vi "1BS3HD_Tidy_v00.vi"(0 "Extras 1SDI":T1={"Error Bit Shift "={"EPR BS"=0, "HD A x"=0, "HD A p"=0, "HD B x"=0, "HD B p"=0, "HD C x"=0, "HD C p"=0}, "I Max value"=20000, "Scan Offset"={"EPR BS"=0.0, "HD A"=0.0, "HD B"=0.0, "HD C"=0.0}, "Scan Ampl.\n     (mV)"={"EPR BS"=0.0, "HD A"=0.0, "HD B"=0.0, "HD C"=0.0}, "Scan-PII thresh"={"EPR BS"=0, "Homodyne A"=0, "Homodyne B"=0, "Homodyne C"=0}, "Re-Scan thresh"={"EPR BS"=1000, "Homodyne A"=1000, "Homodyne B"=1000, "Homodyne C"=0}, "Post-Offset"={"HD A x"=0.0, "HD A p"=0.0, "HD B x"=0.0, "HD B p"=0.0, "HD C x"=0.0, "HD C p"=0.0}}, 5 "EPR BS":T5={"Offset Error"=-0.0003333333333333334, "Gain Error"=1, "P Gain"=25, "P Bit Shift"=-10, "I Bit Shift"=-10, "I Gain"=23, "Lock Threshold"=22, "Lock"=FALSE, "Hold"=FALSE, "Scan Frequency"=17, "Scan Bit Shift"=-4, "Gains +/- "=FALSE, "Pre- Offset Error"=0.0005084745762711861} {"Pre- Offset Error" scale=-0.01..0.01 scale format="%#_5f"; "Scan Frequency" scale=1.0..30.0; "I Gain" scale=0.0..50.0; "P Gain" scale=0.0..50.0; "Offset Error" scale=-0.01..0.01 scale format="%#_5f"}, 7 "Homodyne A":T13={"P Gain"=27, "P Bit Shift"=-8, "I Bit Shift"=-8, "I Gain"=19, "Lock Threshold"=37, "Lock"=FALSE, "Hold"=FALSE, "Scan Frequency"=13, "Scan Bit Shift"=-5, "Gains +/- "=FALSE, "Pre- Offset x"=0.0008474576271186437, "Pre-Offset p"=-0.0023163841807909607, "Gain Error x"=1, "Lock Angle"=0.0, "Gain Error p\n\n"=1} {"Lock Angle" min=-90.0 max=90.0 scale=-90.0..90.0 scale format="%#_2g"; "Pre-Offset p" scale=-0.01..0.01 scale format="%#_5f"; "Pre- Offset x" scale=-0.01..0.01 scale format="%#_5f"; "Scan Frequency" scale=1.0..30.0; "I Gain" scale=0.0..50.0; "P Gain" scale=0.0..50.0}, 9 "Homodyne B":T13={"P Gain"=14, "P Bit Shift"=-8, "I Bit Shift"=-8, "I Gain"=22, "Lock Threshold"=48, "Lock"=FALSE, "Hold"=FALSE, "Scan Frequency"=19, "Scan Bit Shift"=-5, "Gains +/- "=FALSE, "Pre- Offset x"=-0.0016384180790960455, "Pre-Offset p"=-0.002090395480225989, "Gain Error x"=1, "Lock Angle"=15.0, "Gain Error p\n\n"=1} {"Lock Angle" min=-90.0 max=90.0 scale=-90.0..90.0 scale format="%#_2g"; "Pre-Offset p" scale=-0.01..0.01 scale format="%#_5f"; "Pre- Offset x" scale=-0.01..0.01 scale format="%#_5f"; "Scan Frequency" scale=1.0..30.0; "I Gain" scale=0.0..50.0; "P Gain" scale=0.0..50.0}, 11 "Homodyne C":T13={"P Gain"=14, "P Bit Shift"=-8, "I Bit Shift"=-8, "I Gain"=22, "Lock Threshold"=48, "Lock"=FALSE, "Hold"=FALSE, "Scan Frequency"=19, "Scan Bit Shift"=-5, "Gains +/- "=FALSE, "Pre- Offset x"=-0.0016384180790960455, "Pre-Offset p"=-0.002090395480225989, "Gain Error x"=1, "Lock Angle"=15.0, "Gain Error p\n\n"=1} {"Lock Angle" min=-90.0 max=90.0 scale=-90.0..90.0 scale format="%#_2g"; "Pre-Offset p" scale=-0.01..0.01 scale format="%#_5f"; "Pre- Offset x" scale=-0.01..0.01 scale format="%#_5f"; "Scan Frequency" scale=1.0..30.0; "I Gain" scale=0.0..50.0; "P Gain" scale=0.0..50.0}, 12 "Hold All":T16, 14 "Scope+Safety":T18={"Safety First"={"lim reset"=FALSE, "no limit"=FALSE, "pos slew rate * dt"=100, "neg slew rate * dt"=-100, "Count(Ticks)"=0}, "Scope IPs"={"Trigger Direction"=enum."minus-plus", "Trigger Delay (ms)"=0.0, "Aquisition Rate (kHz)"=4000.0, "Trigger Offset (V)"=0.0, "Scale Offset"={"Scaling"={"Error signal"=1, "Output"=1, "DC Monitor"=1, "Threshold"=1}, "Offset"={"Error Signal"=0, "Output"=0, "DC Monitor"=0, "Threshold"=0}}}}) -> (4 "1SDI Control":T15)   [LabVIEW 2013]
doc: "The data structures from the User Interface need are rebundled here to match that of the FPGA_Cavity VI."
uses:
  Strict Type Defs/1BS3HD Control GUI HD.ctl
  Strict Type Defs/PII Gains.ctl
  Strict Type Defs/I16 white control.ctl
  Strict Type Defs/Thresh slider.ctl
  Strict Type Defs/Lock or Hold.ctl
  Strict Type Defs/Scan Freq Slider.ctl
  Strict Type Defs/Gains negative horizontal.ctl
  Strict Type Defs/Slider and display.ctl
  Strict Type Defs/theta 1SDI.ctl
  Strict Type Defs/1BS3HD Control GUI EPR.ctl
  Strict Type Defs/Scope and Safety.ctl
  Strict Type Defs/Safety First.ctl
  Strict Type Defs/Hold All.ctl
  Strict Type Defs/1BS3HD Control dummy.ctl
  Strict Type Defs/1BS3HD Lock Select.ctl
  Strict Type Defs/1BS3HD Extras.ctl
  Strict Type Defs/1BS3HD Double control.ctl
  Strict Type Defs/1BS3HD I16 Control.ctl
panel:
  in  "Lock Select":T4
  in  "1SDI Control dummy":T15
  in  "Safety First":T17
  # "Error Signal"
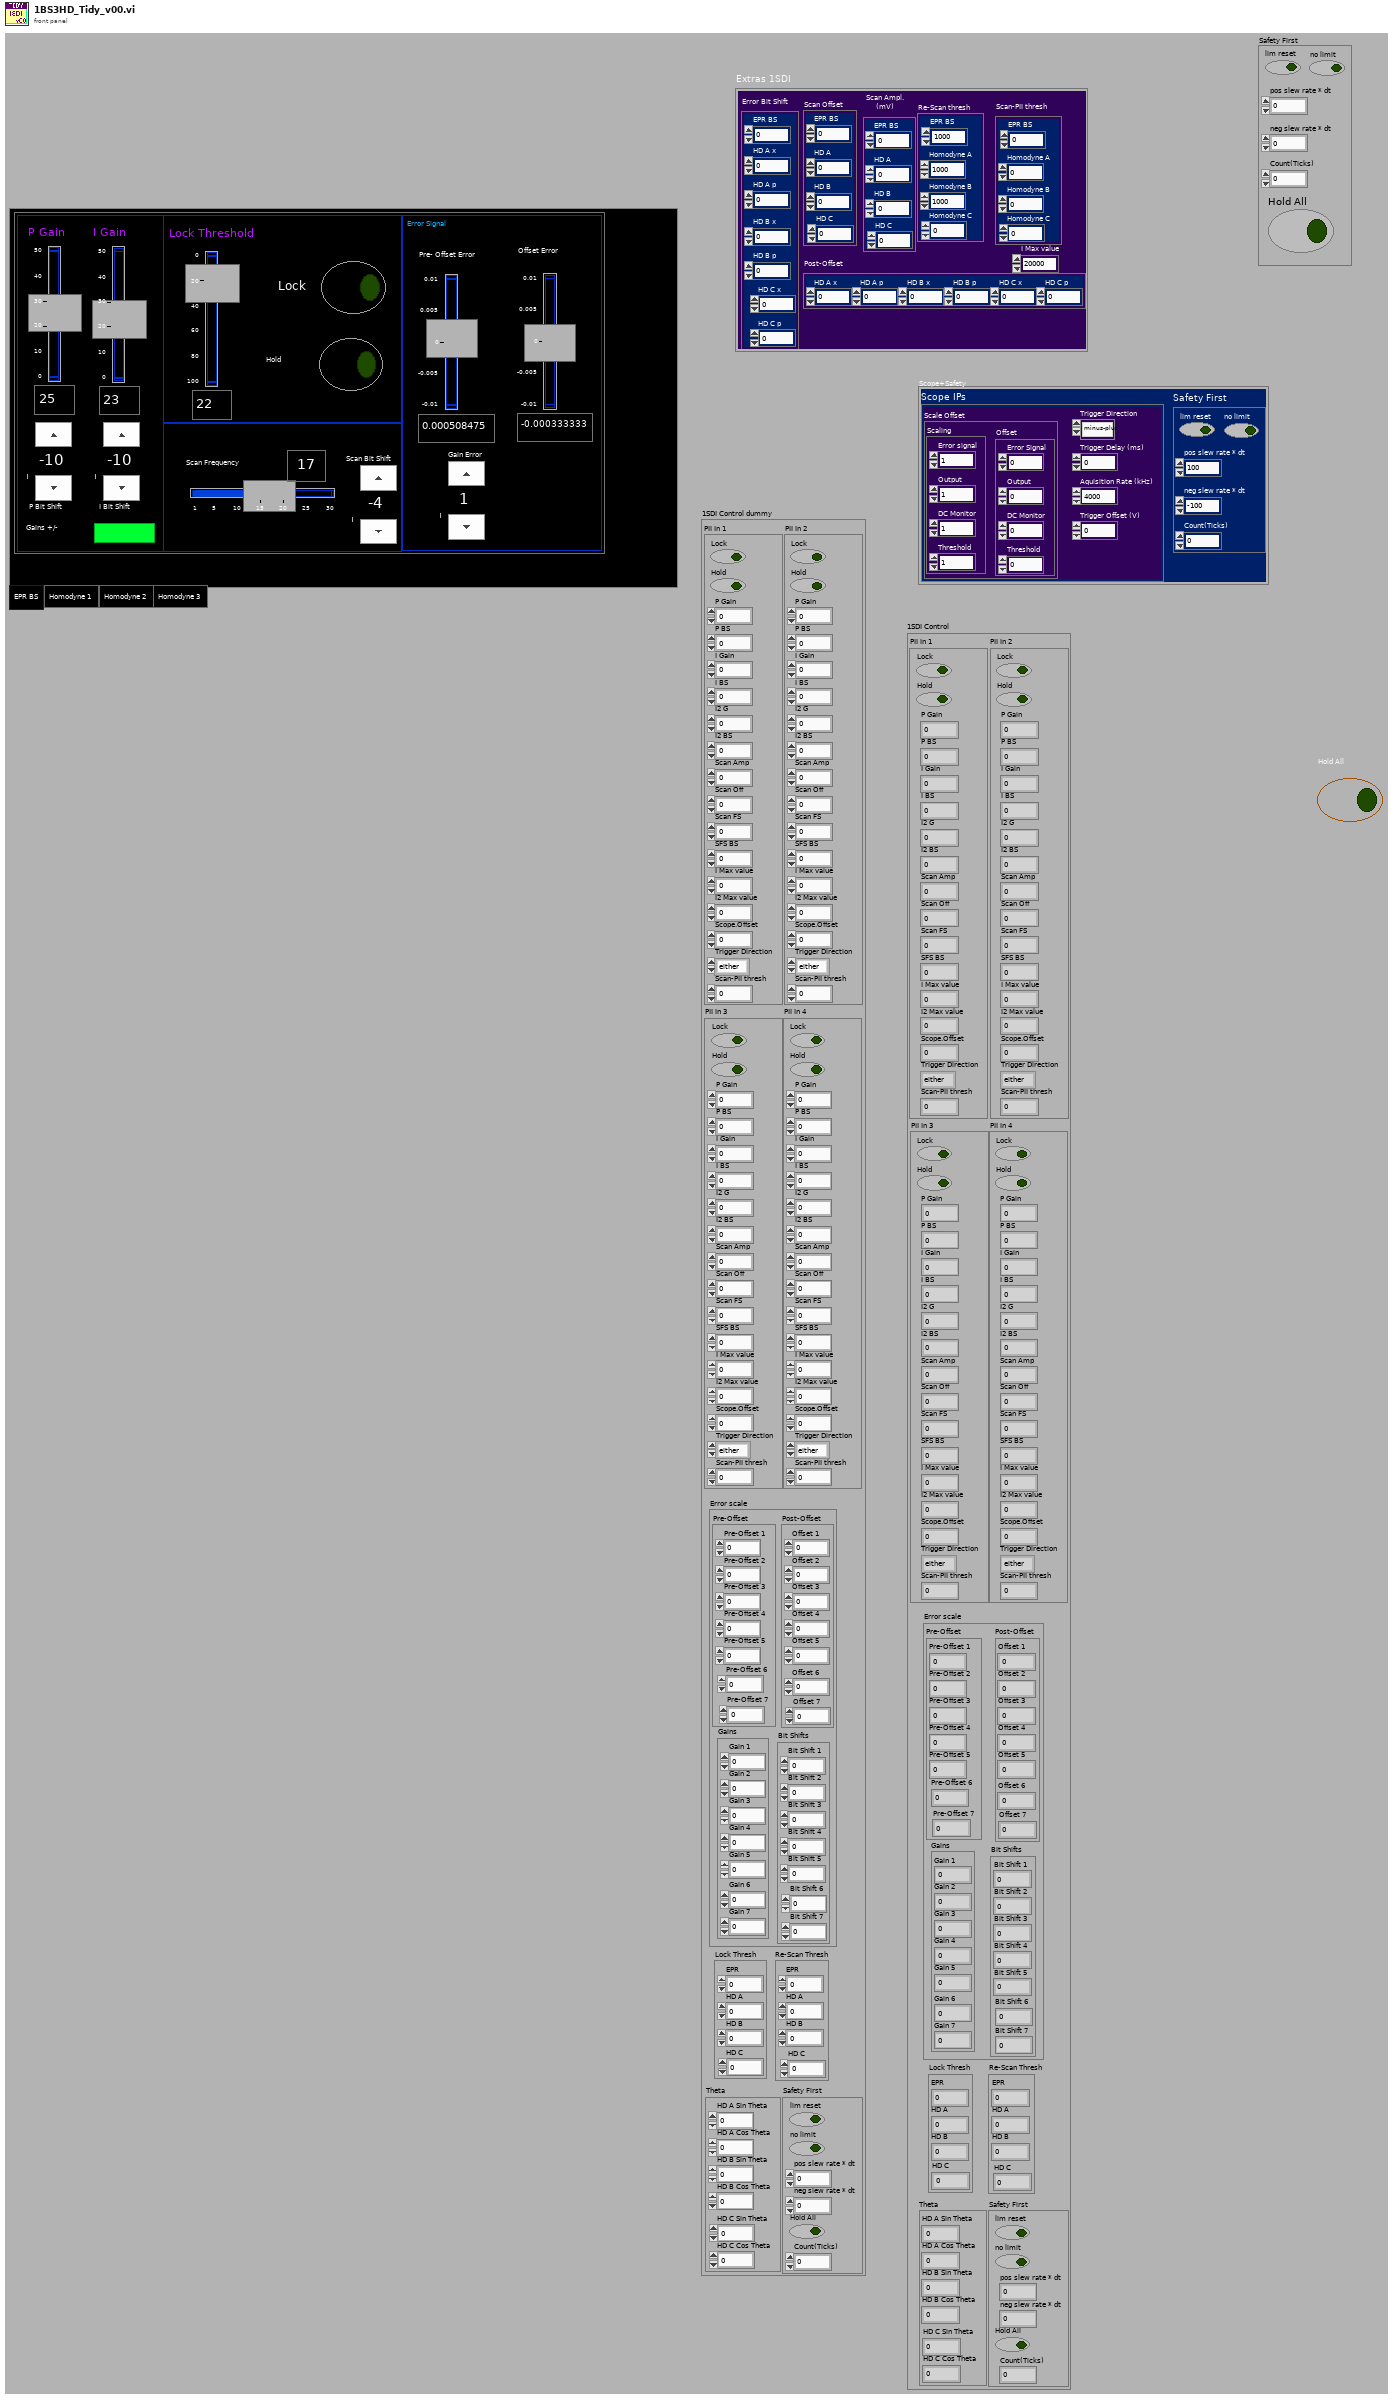
[diagram p1: front panel]
types:
  T1 = typedef "1BS3HD Extras.ctl" = cluster{"Error Bit Shift ":cluster{"EPR BS":i16, "HD A x":i16, "HD A p":i16, "HD B x":i16, "HD B p":i16, "HD C x":i16, "HD C p":i16}, "I Max value":i32, "Scan Offset":T2, "Scan Ampl.\n     (mV)":T2, "Scan-PII thresh":T3, "Re-Scan thresh":T3, "Post-Offset":cluster{"HD A x":dbl, "HD A p":dbl, "HD B x":dbl, "HD B p":dbl, "HD C x":dbl, "HD C p":dbl}}
  T2 = typedef "1BS3HD Double control.ctl" = cluster{"EPR BS":dbl, "HD A":dbl, "HD B":dbl, "HD C":dbl}
  T3 = typedef "1BS3HD I16 Control.ctl" = cluster{"EPR BS":i16, "Homodyne A":i16, "Homodyne B":i16, "Homodyne C":i16}
  T4 = typedef "1BS3HD Lock Select.ctl" = enum32{"EPR BS", "Homodyne 1", "Homodyne 2", "Homodyne 3"}
  T5 = typedef "1BS3HD Control GUI EPR.ctl" = cluster{"Offset Error":T6, "Gain Error":T7, "P Gain":T8, "P Bit Shift":T7, "I Bit Shift":T7, "I Gain":T8, "Lock Threshold":T9, "Lock":T10, "Hold":T10, "Scan Frequency":T11, "Scan Bit Shift":T7, "Gains +/- ":T12, "Pre- Offset Error":T6}
  T6 = typedef "Slider and display.ctl" = dbl
  T7 = typedef "I16 white control.ctl" = i16
  T8 = typedef "PII Gains.ctl" = i32
  T9 = typedef "Thresh slider.ctl" = i16
  T10 = typedef "Lock or Hold.ctl" = bool
  T11 = typedef "Scan Freq Slider.ctl" = u16
  T12 = typedef "Gains negative horizontal.ctl" = bool
  T13 = typedef "1BS3HD Control GUI HD.ctl" = cluster{"P Gain":T8, "P Bit Shift":T7, "I Bit Shift":T7, "I Gain":T8, "Lock Threshold":T9, "Lock":T10, "Hold":T10, "Scan Frequency":T11, "Scan Bit Shift":T7, "Gains +/- ":T12, "Pre- Offset x":T6, "Pre-Offset p":T6, "Gain Error x":T7, "Lock Angle":T14, "Gain Error p\n\n":T7}
  T14 = typedef "theta 1SDI.ctl" = dbl
  T15 = typedef "1BS3HD Control dummy.ctl" = cluster{"PII In 1":cluster{"Lock":bool, "Hold":bool, "P Gain":i32, "P BS":i16, "I Gain":i32, "I BS":i16, "I2 G":i32, "I2 BS":i16, "Scan Amp":i16, "Scan Off":i16, "Scan FS":u16, "SFS BS":i16, "I Max value":i32, "I2 Max value":i32, "Scope.Offset":i16, "Trigger Direction":enum8{"either", "minus-plus", "plus-minus"}, "Scan-PII thresh":i16}, "PII In 2":cluster{"Lock":bool, "Hold":bool, "P Gain":i32, "P BS":i16, "I Gain":i32, "I BS":i16, "I2 G":i32, "I2 BS":i16, "Scan Amp":i16, "Scan Off":i16, "Scan FS":u16, "SFS BS":i16, "I Max value":i32, "I2 Max value":i32, "Scope.Offset":i16, "Trigger Direction":enum8{"either", "minus-plus", "plus-minus"}, "Scan-PII thresh":i16}, "PII In 3":cluster{"Lock":bool, "Hold":bool, "P Gain":i32, "P BS":i16, "I Gain":i32, "I BS":i16, "I2 G":i32, "I2 BS":i16, "Scan Amp":i16, "Scan Off":i16, "Scan FS":u16, "SFS BS":i16, "I Max value":i32, "I2 Max value":i32, "Scope.Offset":i16, "Trigger Direction":enum8{"either", "minus-plus", "plus-minus"}, "Scan-PII thresh":i16}, "Error scale":cluster{"Pre-Offset":cluster{"Pre-Offset 1":i16, "Pre-Offset 2":i16, "Pre-Offset 3":i16, "Pre-Offset 4":i16, "Pre-Offset 5":i16, "Pre-Offset 6":i16, "Pre-Offset 7":i16}, "Post-Offset ":cluster{"Offset 1":i16, "Offset 2":i16, "Offset 3":i16, "Offset 4":i16, "Offset 5":i16, "Offset 6":i16, "Offset 7":i16}, "Gains":cluster{"Gain 1":i16, "Gain 2":i16, "Gain 3":i16, "Gain 4":i16, "Gain 5":i16, "Gain 7":i16, "Gain 6":i16}, "Bit Shifts":cluster{"Bit Shift 1":i16, "Bit Shift 2":i16, "Bit Shift 3":i16, "Bit Shift 4":i16, "Bit Shift 5":i16, "Bit Shift 6":i16, "Bit Shift 7":i16}}, "Lock Thresh":cluster{"EPR":i16, "HD A":i16, "HD B":i16, "HD C":i16}, "Re-Scan Thresh":cluster{"EPR":i16, "HD A":i16, "HD B":i16, "HD C":i16}, "Theta":cluster{"HD A Sin Theta":i32, "HD A Cos Theta":i32, "HD B Sin Theta":i32, "HD B Cos Theta":i32, "HD C Cos Theta":i32, "HD C Sin Theta":i32}, "Safety First":cluster{"lim reset":bool, "no limit":bool, "pos slew rate * dt":i16, "neg slew rate * dt":i16, "Hold All":bool, "Count(Ticks)":u32}, "PII In 4":cluster{"Lock":bool, "Hold":bool, "P Gain":i32, "P BS":i16, "I Gain":i32, "I BS":i16, "I2 G":i32, "I2 BS":i16, "Scan Amp":i16, "Scan Off":i16, "Scan FS":u16, "SFS BS":i16, "I Max value":i32, "I2 Max value":i32, "Scope.Offset":i16, "Trigger Direction":enum8{"either", "minus-plus", "plus-minus"}, "Scan-PII thresh":i16}}
  T16 = typedef "Hold All.ctl" = bool
  T17 = typedef "Safety First.ctl" = cluster{"lim reset":bool, "no limit":bool, "pos slew rate * dt":i16, "neg slew rate * dt":i16, "Hold All":bool, "Count(Ticks)":u32}
  T18 = typedef "Scope and Safety.ctl" = cluster{"Safety First":cluster{"lim reset":bool, "no limit":bool, "pos slew rate * dt":i16, "neg slew rate * dt":i16, "Count(Ticks)":u32}, "Scope IPs":cluster{"Trigger Direction":enum8{"either", "minus-plus", "plus-minus"}, "Trigger Delay (ms)":dbl, "Aquisition Rate (kHz)":dbl, "Trigger Offset (V)":dbl, "Scale Offset":cluster{"Scaling":cluster{"Error signal":i16, "Output":i16, "DC Monitor":i16, "Threshold":i16}, "Offset":cluster{"Error Signal":i16, "Output":i16, "DC Monitor":i16, "Threshold":i16}}}}
  T19 = enum32{"OPO A", "OPO B", "Mode Cleaner", "Doubler", "パラメ OPO A", "パラメ OPO B", "EPR Beamsplitter", "Graph Beamsplitter", "Homodyne A", "Homodyne B"}
  T20 = cluster{"lim reset":bool, "no limit":bool, "pos slew rate * dt":i16, "neg slew rate * dt":i16, "Count(Ticks)":u32}
  T21 = typedef "Extras PII 1SDI HD.ctl" = cluster{"Error Bit Shift p":i16, "Scan Offset":dbl, "Scan Amplitude":dbl, "Scan-PII thresh":i16, "Re-Scan Thresh":i16, "I Max value":i32, "Trigger Direction":enum8{"either", "minus-plus", "plus-minus"}, "Trigger Offset (V)":dbl, "Error Bit Shift x":i16, "Post-Offset p":dbl, "Post-Offset x":dbl}
  T22 = typedef "Extras PII 1SDI.ctl" = cluster{"Error Bit Shift":i16, "Scan Offset":dbl, "Scan Amplitude":dbl, "Scan-PII thresh":i16, "Re-Scan Thresh":i16, "I Max value":i32, "Trigger Direction":enum8{"either", "minus-plus", "plus-minus"}, "Trigger Offset (V)":dbl}
  T23 = typedef "PII and Error Graph.ctl" = cluster{"Error individual":T24, "PII cavity":T25, "Lock Thresh":i16, "Re-Scan Thresh":i16}
  T24 = typedef "Errors Converted Graph.ctl" = cluster{"Error Pre Offset":i16, "Error Offset":i16, "Error Gain":i16, "Error Bit Shift":i16}
  T25 = typedef "PII individual.ctl" = cluster{"Lock":bool, "Hold":bool, "P Gain":i32, "P BS":i16, "I Gain":i32, "I BS":i16, "I2 G":i32, "I2 BS":i16, "Scan Amp":i16, "Scan Off":i16, "Scan FS":u16, "SFS BS":i16, "I Max value":i32, "I2 Max value":i32, "Scope.Offset":i16, "Trigger Direction":enum8{"either", "minus-plus", "plus-minus"}, "Scan-PII thresh":i16}
  T26 = typedef "PII and Error Graph HD.ctl" = cluster{"Error individual":T27, "PII cavity":T25, "Lock Thresh":i16, "Re-Scan Thresh":i16, "Sin Theta":i32, "Cos Theta":i32}
  T27 = typedef "Errors Converted Graph HD.ctl" = cluster{"Error Pre Offset x":i16, "Error Offset x":i16, "Error Gain x":i16, "Error Bit Shift x":i16, "Error Pre Offset p":i16, "Error Offset p":i16, "Error Gain p":i16, "Error Bit Shift p":i16}
  T28 = typedef "1BS3HD Theta.ctl" = cluster{"HD A Sin Theta":i32, "HD A Cos Theta":i32, "HD B Sin Theta":i32, "HD B Cos Theta":i32, "HD C Sin Theta":i32, "HD C Cos Theta":i32}
  T29 = typedef "1BS3HD Lock Thresh.ctl" = cluster{"EPR":i16, "HD A":i16, "HD B":i16, "HD C":i16}
  T30 = typedef "1BS3HD Error Scale.ctl" = cluster{"Pre-Offset":cluster{"Pre-Offset 1":i16, "Pre-Offset 2":i16, "Pre-Offset 3":i16, "Pre-Offset 4":i16, "Pre-Offset 5":i16, "Pre-Offset 6":i16, "Pre-Offset 7":i16}, "Post-Offset ":cluster{"Offset 1":i16, "Offset 2":i16, "Offset 3":i16, "Offset 4":i16, "Offset 5":i16, "Offset 6":i16, "Offset 7":i16}, "Gains":cluster{"Gain 1":i16, "Gain 2":i16, "Gain 3":i16, "Gain 4":i16, "Gain 5":i16, "Gain 6":i16, "Gain 7":i16}, "Bit Shifts":cluster{"Bit Shift 1":i16, "Bit Shift 2":i16, "Bit Shift 3":i16, "Bit Shift 4":i16, "Bit Shift 5":i16, "Bit Shift 6":i16, "Bit Shift 7":i16}}
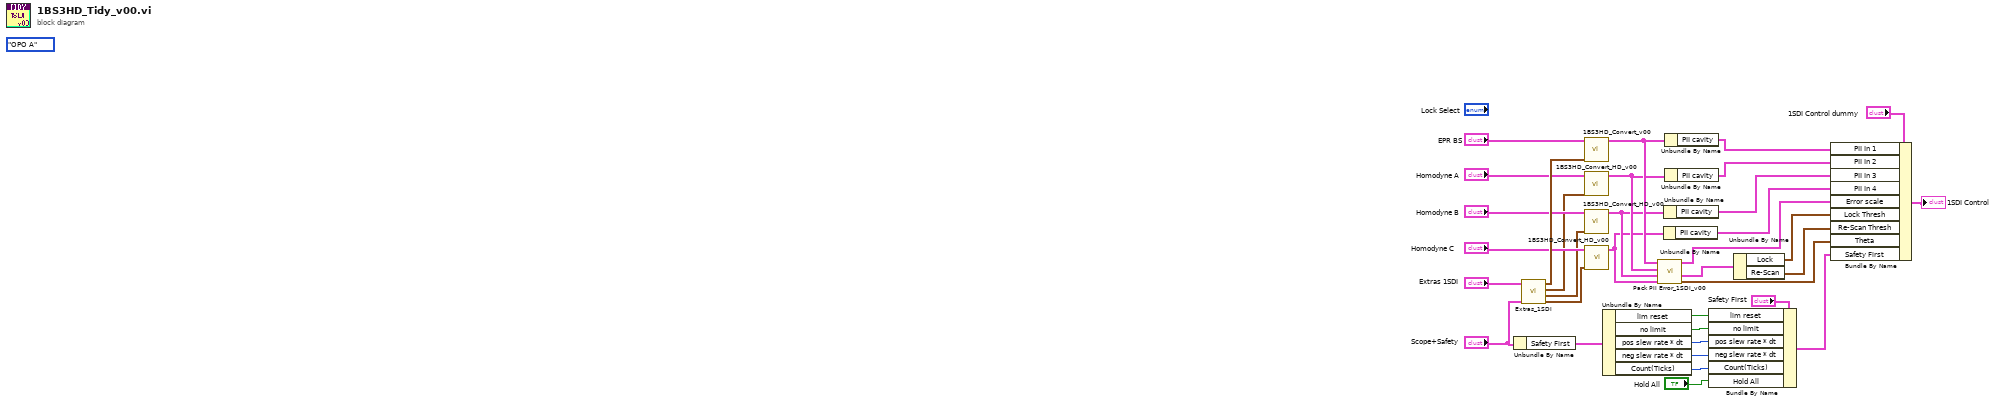
[diagram p0: block diagram]
diagram:
  (unwired) T19."OPO A" ("Tab Control")
  n1 = Unbundle By Name("Scope+Safety") -> ("Safety First"=w17:T20)
  n2 = call "Extras_1SDI.vi"("Scope+Safety"="Scope+Safety", "Extras 1SDI"="Extras 1SDI") -> ("Extras Homodyne C"=w5:T21, "Extras Homodyne B"=w6:T21, "Extras Homodyne A"=w7:T21, "Extras EPR BS"=w25:T22)  [unwired: 6 in]
  n3 = call "1BS3HD_Convert_v00.vi"("Extras PII"=w25, "PII Control"="EPR BS") -> ("PII+Error"=w34:T23)  [unwired: 9 in]
  n4 = call "1BS3HD_Convert_HD_v00.vi"("Extras Homodyne"=w7, "PII Control"="Homodyne A") -> ("PII+Error"=w4:T26)  [unwired: 9 in]
  n5 = call "1BS3HD_Convert_HD_v00.vi"("Extras Homodyne"=w6, "PII Control"="Homodyne B") -> ("PII+Error"=w3:T26)  [unwired: 9 in]
  n6 = call "1BS3HD_Convert_HD_v00.vi"("Extras Homodyne"=w5, "PII Control"="Homodyne C") -> ("PII+Error"=w2:T26)  [unwired: 9 in]
  n7 = Unbundle By Name(w17) -> ("lim reset"=w32:bool, "no limit"=w31:bool, "pos slew rate * dt"=w30:i16, "neg slew rate * dt"=w29:i16, "Count(Ticks)"=w28:u32)
  n8 = call "Pack PII Error_1SDI_v00.vi"("PII+Error HD C"=w2, "PII+Error HD B"=w3, "PII+Error HD A"=w4, "PII+Error EPR BS"=w34) -> ("Theta"=w21:T28, "Thresholds"=w22:cluster{"Lock":T29, "Re-Scan":T29}, "Error packed"=w9:T30)  [unwired: 5 in]
  n9 = Unbundle By Name(w2) -> ("PII cavity"=w1:T25)
  n10 = Unbundle By Name(w3) -> ("PII cavity"=w10:T25)
  n11 = Unbundle By Name(w34) -> ("PII cavity"=w12:T25)
  n12 = Unbundle By Name(w4) -> ("PII cavity"=w11:T25)
  n13 = Bundle By Name(cluster="Safety First", "lim reset"=w32, "no limit"=w31, "pos slew rate * dt"=w30, "neg slew rate * dt"=w29, "Count(Ticks)"=w28, "Hold All"="Hold All") -> (w26:T17)
  n14 = Unbundle By Name(w22) -> ("Lock"=w24:T29, "Re-Scan"=w23:T29)
  n15 = Bundle By Name(cluster="1SDI Control dummy", "PII In 1"=w12, "PII In 2"=w11, "PII In 3"=w10, "PII In 4"=w1, "Error scale"=w9, "Lock Thresh"=w24, "Re-Scan Thresh"=w23, "Theta"=w21, "Safety First"=w26) -> (→"1SDI Control":T15)
